vi "Configure Retransmit Output.vi"(0 "VISA resource name":refnum<visa-resource-name>, 1 "Unit Address (1)":i16=1, 2 "Analog Range (0: 4 to 20 mA)":u16(ring) items=["4 to 20 mA", "0 to 20 mA", "0 to 5 V", "1 to 5 V", "0 to 10 V"], 3 "Retransmit Source (0: Input 1)":u16(ring) items=["Input 1", "Input 2", "Input 3", "Set Point 1", "Set Point 2", "Channel 1 Power", "Channel 2 Power"], 5 "Retransmit Output (1)":i16=1, 7 "Low Scale (-19999.0)":dbl=-19999.0 format="%.2f", 9 "High Scale (30000.0)":dbl=30000.0 format="%.2f", 11 "error in (no error)":errorcluster {"code" format="%.0x"}, 12 "Scale Offset (0.0)":dbl format="%.2f") -> (4 "VISA resource name out":refnum<visa-resource-name>, 15 "error out":errorcluster {"code" format="%.0x"})   [LabVIEW 2010]
doc: "This VI configures retransmit output."
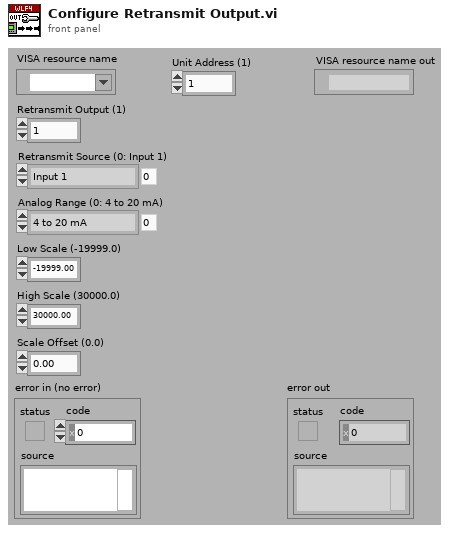
[diagram p1: front panel]
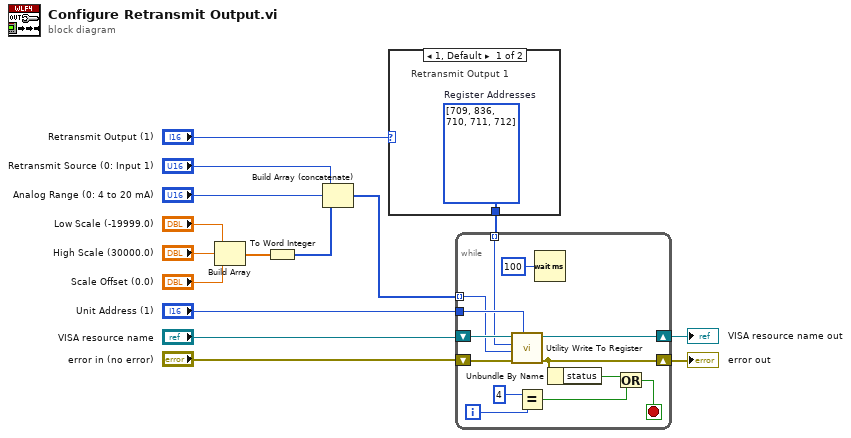
[diagram p0: block diagram]
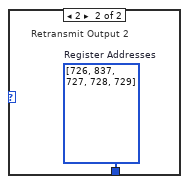
[diagram p2: hidden frame]
diagram:
  n1 = Build Array("Low Scale (-19999.0)", "High Scale (30000.0)", "Scale Offset (0.0)") -> (w3:dbl[])
  n2 = To Word Integer(number=w3) -> (16bit integer=w2:i16[])
  n3 = Build Array (concatenate)("Retransmit Source (0: Input 1)", "Analog Range (0: 4 to 20 mA)", w2) -> (w1:u16[])
  n4 = case shown="1, Default" "Retransmit Output (1)" {
    tunnel: [w16 w17] -> w12
    frame 1, Default {
      w16 = i32[] [709, 836, 710, 711, 712]  # Register Addresses
      # "Retransmit Output 1"
    }
    frame 2 {
      w17 = i32[] [726, 837, 727, 728, 729]  # Register Addresses
      # "Retransmit Output 2"
    }
  }
  n5 = while {
    tunnel: "Unit Address (1)" -> [w30]
    shift-right: [w27] -> w15
    shift-left: "VISA resource name" -> [w29]
    shift-right: [w23] -> w14
    shift-left: "error in (no error)" -> [w28]
    tunnel: w12 -> [w25] mode=indexing
    tunnel: w1 -> [w24] mode=indexing
    i -> [w20]
    stop <- w22 stop-if-true
    n6 = call "Utility Write To Register.vi"("Unit Address (1)"=w30, "error in (no error)"=w28, "Data (0)"=w24, "Register Address (0)"=w25, "VISA resource name"=w29) -> ("error out"=w23:errorcluster, "VISA resource name out"=w27:refnum<visa-resource-name>)  [unwired: 5 in]
    n7 = Equal?(x=4, y=w20) -> (x = y?=w18:bool)
    n8 = Wait (ms)(milliseconds to wait=u32 100) -> ()  [unwired: 1 out]
    n9 = Unbundle By Name(w23) -> ("status"=w21:bool)
    n10 = Or(x=w21, y=w18) -> (x .or. y?=w22:bool)
  }
  "error out" <- w14
  "VISA resource name out" <- w15
